vi "svfa_Convert to One-Sided FFT Spectrum.vi"(0 "two-sided FFT spectrum":cdb[](array[numeric]) format="%.2f") -> (1 "one-sided FFT spectrum":cdb[](array[numeric]) format="%.2f", 2 "block size":dbl format="%.2f")   [LabVIEW 2017]
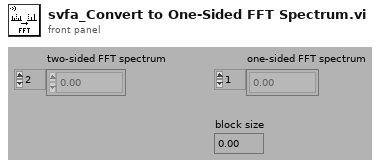
[diagram p1: front panel]
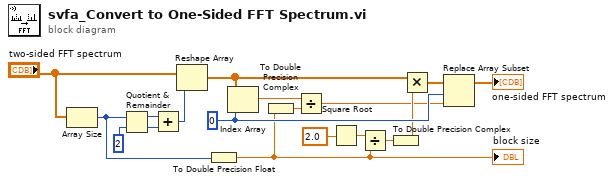
[diagram p0: block diagram]
diagram:
  w16 = 0
  n1 = Array Size(array="two-sided FFT spectrum") -> (size(s)=w6:i32)
  n2 = Quotient & Remainder(x=w6, y=2) -> (x-y*floor(x/y)=w14:i32, floor(x/y)=w13:i32)
  n3 = Add(x=w14, y=w13) -> (x+y=w12:i32)
  n4 = Reshape Array("two-sided FFT spectrum", w12) -> (w4:cdb[])
  n5 = To Double Precision Float(number=w6) -> (double precision float=w1:dbl)
  "block size" <- w1
  n6 = Index Array(array=w4, index=w16) -> (element=w2:cdb)
  n7 = To Double Precision Complex(1:w1) -> (0:w3:cdb)
  n8 = Divide(x=w2, y=w3) -> (x/y=w5:cdb)
  n9 = Square Root(x=2.0) -> (sqrt(x)=w8:dbl)
  n10 = Divide(x=w8, y=w1) -> (x/y=w7:dbl)
  n11 = To Double Precision Complex(1:w7) -> (0:w11:cdb)
  n12 = Multiply(x=w4, y=w11) -> (x*y=w9:cdb[])
  n13 = Replace Array Subset(array=w9, new element=w5, index=w16) -> (→"one-sided FFT spectrum":cdb[])
